vi "BuildErrorSource.vi"(8 "error in":errorcluster, 10 "status code":i32=1, 11 "extended error info":string) -> (0 "error out":errorcluster)   [LabVIEW 2013, in "fileversion.lvlib"]
doc: "This subVI reads in an error description and creates a custom error code for that description between 5000 and 9000. The result should be fairly unique."
uses:
  fileversion.lvlib
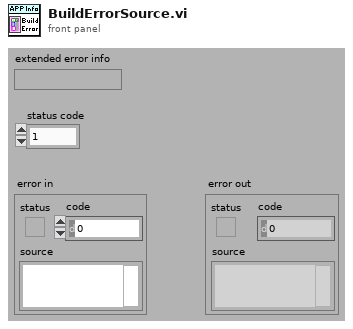
[diagram p1: front panel]
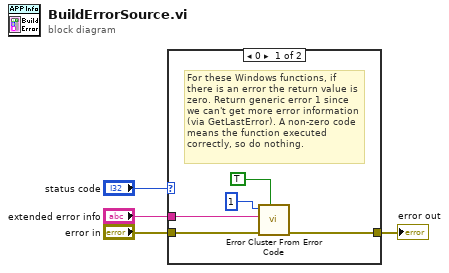
[diagram p0: block diagram]
diagram:
  n1 = case shown="0" "status code" {
    tunnel: "error in" -> [w9 w10]
    tunnel: [w8 w10] -> w3
    tunnel: "extended error info" -> [w7 _]
    frame 0 {
      # "For these Windows functions, if there is an error the return value is zero. Return generic error 1 since we can't get more error information (via GetLastError). A non-zero code means the function executed correctly, so do nothing."
      n2 = call <vilib>:"Error Cluster From Error Code.vi"("show call chain? (False)"=TRUE, "error in (no error)"=w9, "error message (\"\")"=w7, "error code (0)"=1 ("t")) -> ("error out"=w8:errorcluster)  [unwired: 5 in]
    }
    frame Default {
    }
  }
  "error out" <- w3
